vi "KalmanFilter_Correct.vi"(9 "Y":T1, 10 "U":T1, 11 "in KalmanFilter":T2) -> (0 "Error":bool, 3 "out KalmanFilter":T2)   [LabVIEW 2019, in "Trajectory_Library.lvlib"]
doc: "Correct the state estimate x-hat using the measurements in y.\n \nInputs:\n - inKalmanFIlter -- filter data cluster\n - u -- Same control input used in the last predict step.\n - y -- Measurement vector.\n\nOutputs:\n - outKalmanFilter -- updated filter data cluster\n - error -- If true, an error occured"
uses:
  Trajectory_Library.lvlib
  <vilib>/Analysis/NI_AALBase.lvlib
  <vilib>/Analysis/baseanly.llb/Real A x B.vi
  <vilib>/Analysis/Matrix/NI_Matrix.lvlib
  <vilib>/Analysis/Matrix/Numeric/Add/Add - RM,RM.vi
  <vilib>/Analysis/Matrix/Numeric/Subtract/Subtract - RM,RM.vi
  <vilib>/Analysis/Matrix/Datatypes/RealMatrix.ctl
  TypeDef/LINEAR_SYSTEM.ctl
  TypeDef/KALMAN_FILTER.ctl
panel:
  # "<Inputs,1>"
  # "<Outputs,1>"
  # "Steady State Gain  \n<States,Outputs>"
  # "State Estimate <Statess,1>"
  # "<States,States>"
  # "<States,Inputs>"
  # "<Outputs,States>"
  # "<Outputs,Inputs>"
  # "Steady State Gain  \n<States,Outputs>"
  # "State Estimate <Statess,1>"
  # "<States,States>"
  # "<States,Inputs>"
  # "<Outputs,States>"
  # "<Outputs,Inputs>"
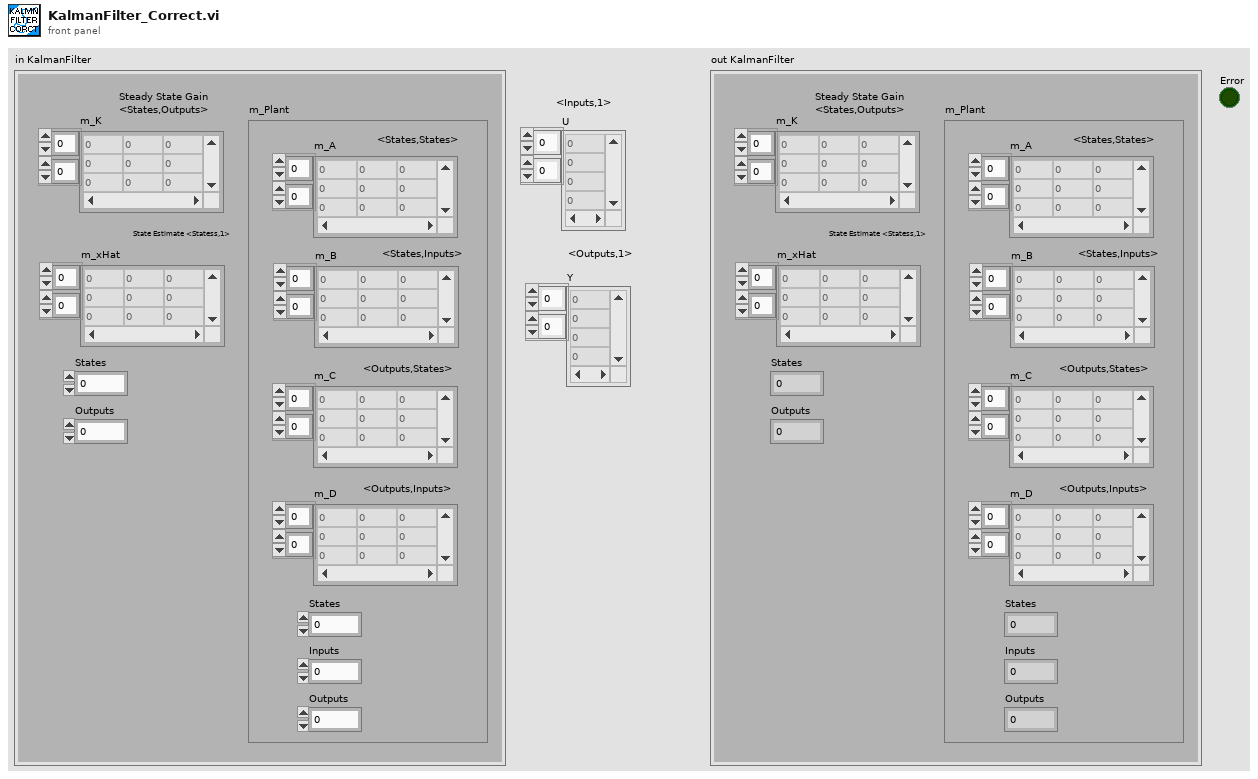
[diagram p1: front panel]
types:
  T1 = typedef "NI_Matrix.lvlib/RealMatrix.ctl" = dbl[][]
  T2 = typedef "Trajectory_Library.lvlib/KALMAN_FILTER.ctl" = cluster{"m_K":T1, "m_xHat":T1, "States":i32, "Outputs":i32, "m_Plant":T3}
  T3 = typedef "Trajectory_Library.lvlib/LINEAR_SYSTEM.ctl" = cluster{"m_A":T1, "m_B":T1, "m_C":T1, "m_D":T1, "States":i32, "Inputs":i32, "Outputs":i32}
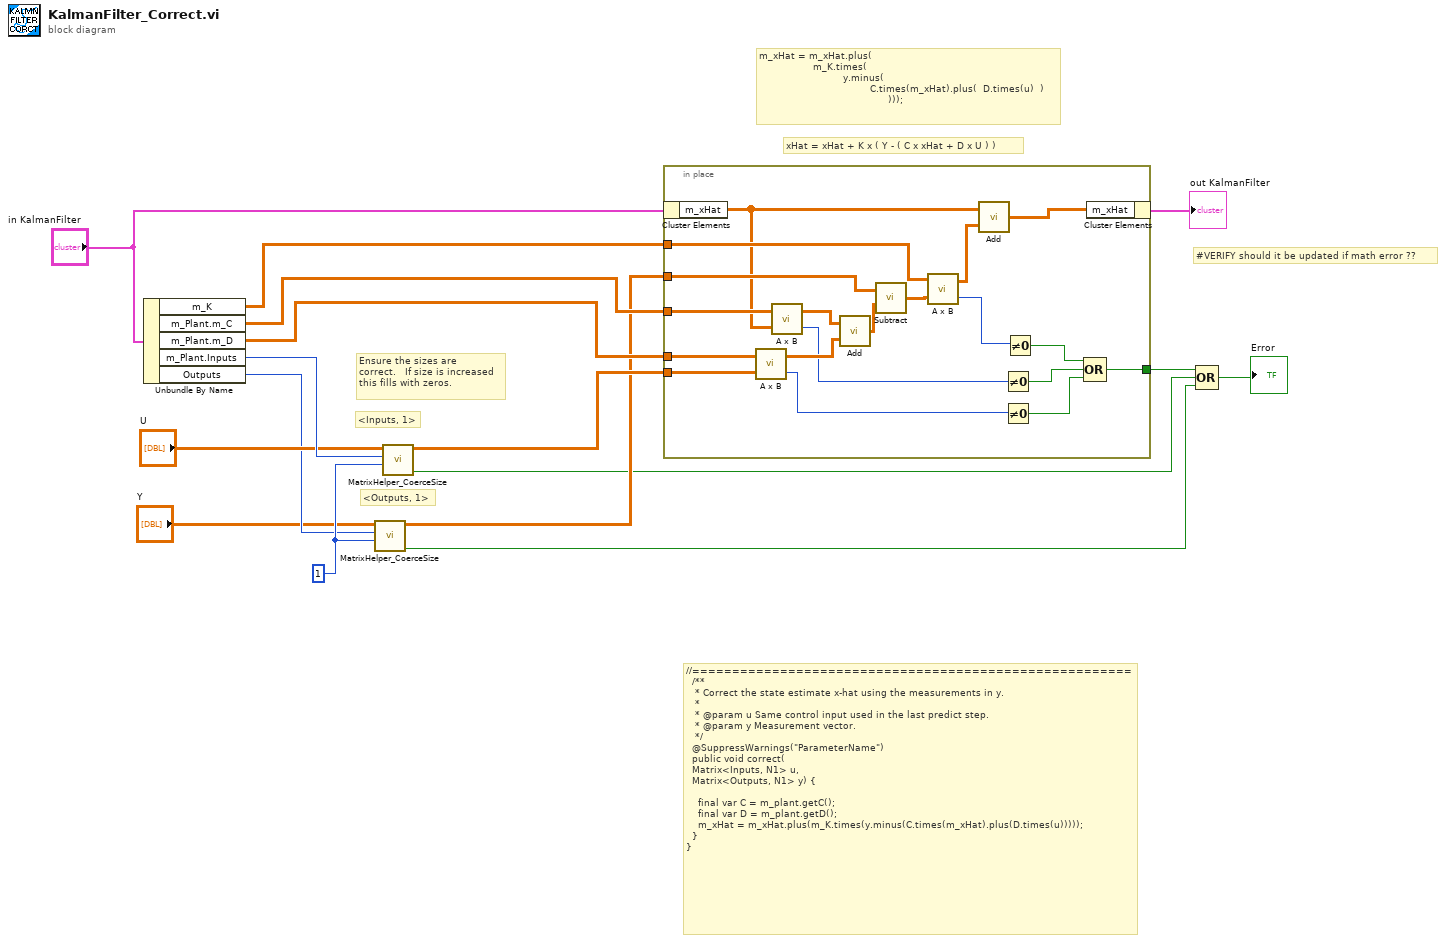
[diagram p0: block diagram]
diagram:
  w8 = 1 ("y")
  # "#VERIFY should it be updated if math error ??"
  # "xHat = xHat + K x ( Y - ( C x xHat + D x U ) )"
  # "m_xHat = m_xHat.plus(\n                  m_K.times(\n                            y.minus(\n                                     C.times(m_xHat).plus(  D.times(u)  )\n                                           )));"
  # "<Outputs, 1>"
  # "<Inputs, 1>"
  # "//=======================================================\n  /**\n   * Correct the state estimate x-hat using the measurements in y.\n   *\n   * @param u Same control input used in the last predict step.\n   * @param y Measurement vector.\n   */\n  @SuppressWarnings(\"ParameterName\")\n  public void correct(\n\t\tMatrix<Inputs, N1> u, \n\t\tMatrix<Outputs, N1> y) {\n\n    final var C = m_plant.getC();\n    final var D = m_plant.getD();\n    m_xHat = m_xHat.plus(m_K.times(y.minus(C.times(m_xHat).plus(D.times(u)))));\n  }\n}"
  # "Ensure the sizes are\ncorrect.   If size is increased \nthis fills with zeros."
  n1 = Unbundle By Name("in KalmanFilter") -> ("m_K"=w13:T1, "m_Plant.m_C"=w14:T1, "m_Plant.m_D"=w15:T1, "m_Plant.Inputs"=w11:i32, "Outputs"=w7:i32)
  n2 = call "MatrixHelper_CoerceSize.vi"("Columns"=w8, "Rows"=w7, "input matrix"="Y") -> ("Coerced"=w2:bool, "output matrix"=w5:T1)  [unwired: 7 in]
  n3 = call "MatrixHelper_CoerceSize.vi"("Columns"=w8, "Rows"=w11, "input matrix"="U") -> ("Coerced"=w3:bool, "output matrix"=w9:T1)  [unwired: 7 in]
  n4 = in-place {
    in-place-border: w15 -> [w35]
    in-place-border: w9 -> [w34]
    in-place-border: w14 -> [w33]
    in-place-border: w5 -> [w29]
    in-place-border: w13 -> [w27]
    in-place-border: [w17] -> w4
    n5 = in-place-cluster #1("in KalmanFilter") -> ("m_xHat"=w25:T1)
    n6 = call-poly <vilib>:"A x B.vi"("B"=w34, "A"=w35) -> ("error"=w22:i32, "A x B"=w31:T1)
    n7 = call-poly <vilib>:"A x B.vi"("B"=w25, "A"=w33) -> ("error"=w23:i32, "A x B"=w32:T1)
    n8 = call-poly <vilib>:"Add.vi"("Real Matrix B"=w31, "Real Matrix A"=w32) -> ("A + B"=w30:T1)
    n9 = call-poly <vilib>:"Subtract.vi"("Real Matrix B"=w30, "Real Matrix A"=w29) -> ("A - B"=w28:T1)
    n10 = call-poly <vilib>:"A x B.vi"("B"=w28, "A"=w27) -> ("error"=w21:i32, "A x B"=w26:T1)
    n11 = call-poly <vilib>:"Add.vi"("Real Matrix B"=w26, "Real Matrix A"=w25) -> ("A + B"=w24:T1)
    n12 = Not Equal To 0?(x=w23) -> (x != 0?=w19:bool)
    n13 = Not Equal To 0?(x=w22) -> (x != 0?=w18:bool)
    n14 = Not Equal To 0?(x=w21) -> (x != 0?=w20:bool)
    n15 = Compound Arithmetic op=OR(w20, w19, w18) -> (w17:bool)
    n16 = in-place-cluster #1("m_xHat"=w24) -> (→"out KalmanFilter":T2)
  }
  n17 = Compound Arithmetic op=OR(w4, w3, w2) -> (→"Error":bool)
